vi "VescTest.vi"() -> ()   [LabVIEW 2019]
uses:
  <vilib>/Instr/_visa.llb/VISA Configure Serial Port (Instr).vi
panel:
  out "return count":u32
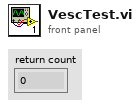
[diagram p1: front panel]
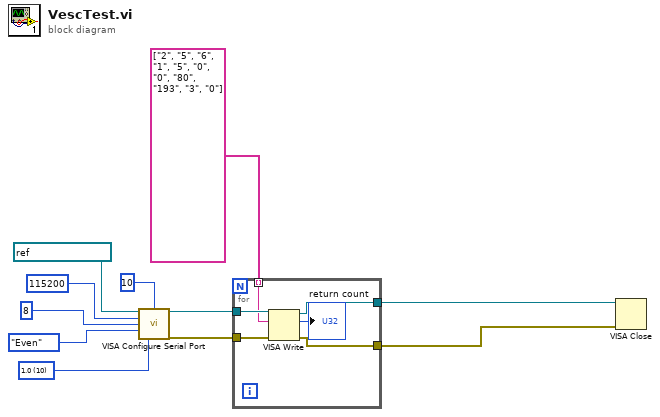
[diagram p0: block diagram]
diagram:
  w7 = u16 10 items=["1.0"=10, "1.5"=15, "2.0"=20] ("stop bits (10: 1 bit)")
  n1 = call-poly "VISA Configure Serial Port"("VISA resource name"=refnum<visa-resource-name> "ASRL2::INSTR", "termination char\n(0xA = '\\n' = LF)"=u8 10 ("termination char\n(0xA = '\\n' = LF)"), "baud rate (9600)"=u32 115200, "data bits (8)"=u16 8, "parity (0:none)"=enum16{"None", "Odd", "Even", "Mark", "Space"}."Even", "stop bits (10: 1 bit)"=w7) -> ("VISA resource name out"=w5:refnum<visa-resource-name>, "error out"=w1:errorcluster)  [unwired: 8 in]
  n2 = for {
    tunnel: w5 -> [w17]
    tunnel: string[] ["2", "5", "6", "1", "5", "0", "0", "80", "193", "3", "0"] -> [w16] mode=indexing
    tunnel: [w15] -> w3
    tunnel: [w13] -> w2
    tunnel: w1 -> [w12]
    n3 = VISA Write(VISA resource name=w17, write buffer=w16, error in (no error)=w12) -> (VISA resource name out=w15:refnum<visa-resource-name>, return count=→"return count":u32, error out=w13:errorcluster)
  }
  n4 = VISA Close(VISA resource name=w3, error in (no error)=w2) -> ()  [unwired: 1 out]
